vi "Calculate Jacobian.vi"(7 "Error Evaluation":T6, 9 "Validation Set":T2[](array[typedef]), 10 "Teaching Set":T2[](array[typedef]), 11 "Neural Network In":T4) -> (2 "Total Error":dbl, 3 "Jacobian":T1[][](array[typedef]))   [LabVIEW 2011, in "Super Simple Neural Network.lvlib"]
uses:
  Super Simple Neural Network.lvlib
  Types/Error Evaluation.ctl
  Types/2D Array.ctl
  Types/Neural Network.ctl
  Types/1D Array.ctl
  Types/Teaching Vector.ctl
  Types/Scaling Info.ctl
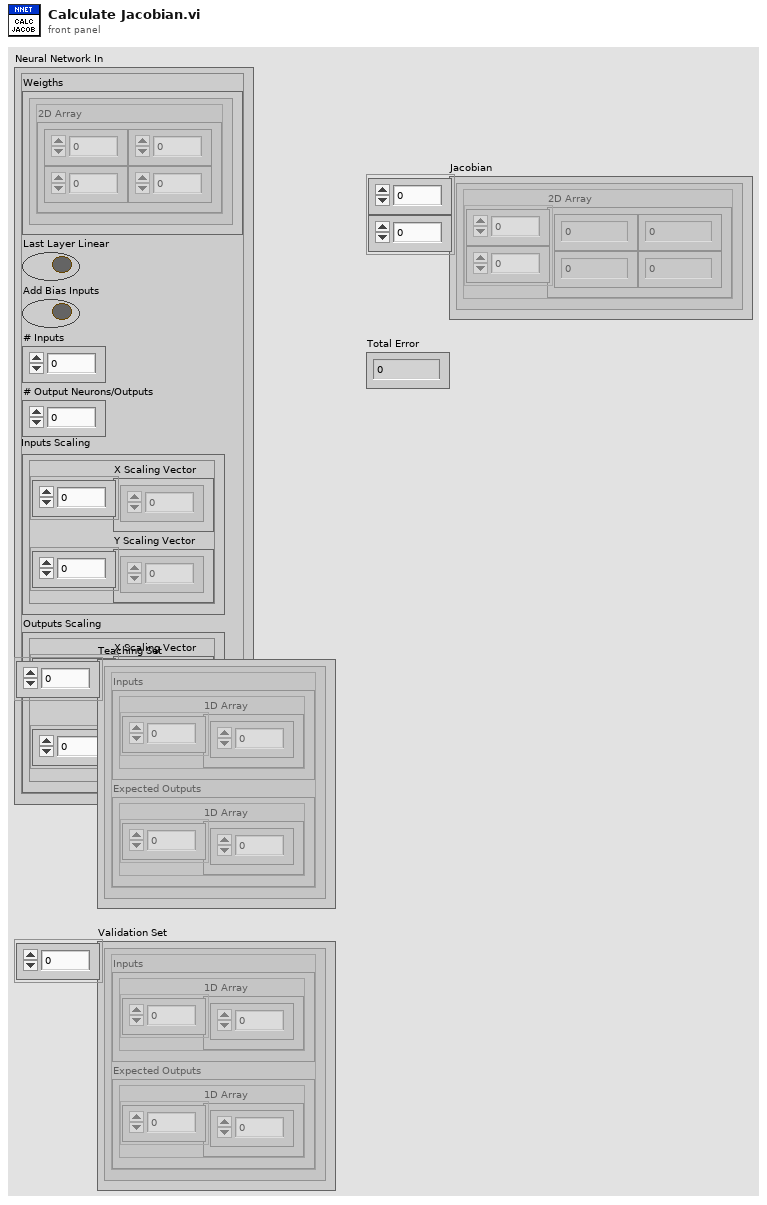
[diagram p1: front panel]
types:
  T1 = typedef "Super Simple Neural Network.lvlib/2D Array.ctl" = cluster{"2D Array":dbl[][]}
  T2 = typedef "Super Simple Neural Network.lvlib/Teaching Vector.ctl" = cluster{"Inputs":T3, "Expected Outputs":T3}
  T3 = typedef "Super Simple Neural Network.lvlib/1D Array.ctl" = cluster{"1D Array":dbl[]}
  T4 = typedef "Super Simple Neural Network.lvlib/Neural Network.ctl" = cluster{"Weigths":T1[], "Last Layer Linear":bool, "Add Bias Inputs":bool, "# Inputs":u32, "# Output Neurons/Outputs":u32, "Inputs Scaling":T5, "Outputs Scaling":T5}
  T5 = typedef "Super Simple Neural Network.lvlib/Scaling Info.ctl" = cluster{"X Scaling Vector":dbl[], "Y Scaling Vector":dbl[]}
  T6 = typedef "Super Simple Neural Network.lvlib/Error Evaluation.ctl" = enum16{"Over Both Sets", "Over Validation Set", "Over Teaching Set"}
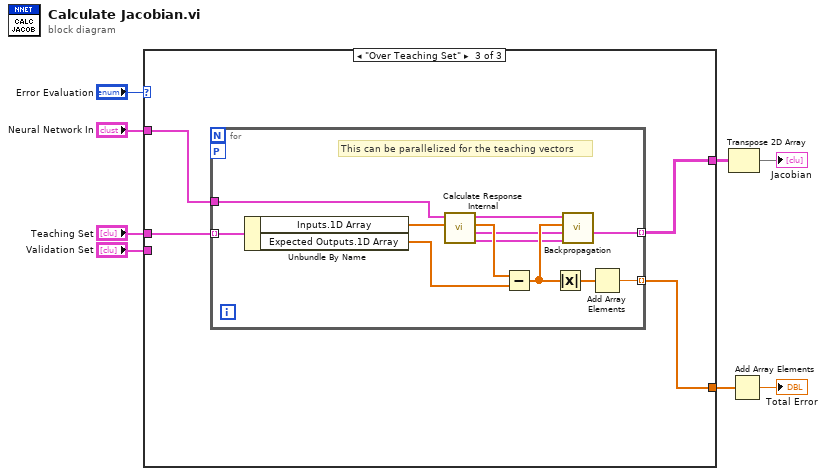
[diagram p0: block diagram]
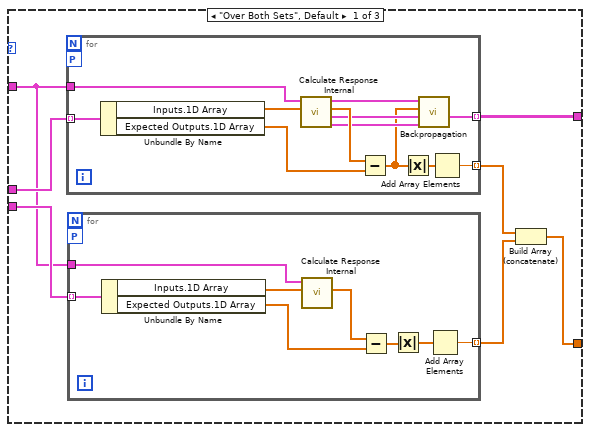
[diagram p2: hidden frame]
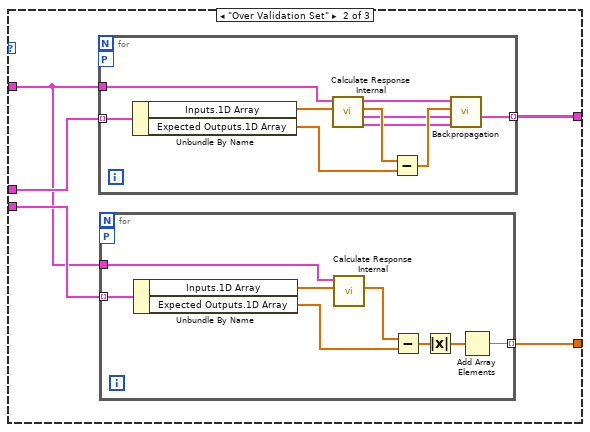
[diagram p3: hidden frame]
diagram:
  n1 = case shown="\"Over Teaching Set\"" "Error Evaluation" {
    tunnel: "Neural Network In" -> [w12 w37 w62]
    tunnel: "Teaching Set" -> [w15 w40 w61]
    tunnel: [w9 w36 w60] -> w1
    tunnel: [w14 w39 w59] -> w3
    tunnel: "Validation Set" -> [w13 w38 _]
    frame "Over Both Sets", Default {
      n2 = for {
        tunnel: w15 -> [w35] mode=indexing
        tunnel: [w27] -> w14 mode=indexing
        workers-P: _ -> [_]
        tunnel: w12 -> [w31]
        tunnel: [w24] -> w11 mode=indexing
        n3 = Unbundle By Name(w35) -> ("Inputs.1D Array"=w33:dbl[], "Expected Outputs.1D Array"=w34:dbl[])
        n4 = call "Calculate Response Internal.vi"("Inputs"=w33, "Neural Network In"=w31) -> ("All Inputs"=w28:T3[], "Derrivatives"=w29:T3[], "Outputs"=w32:dbl[], "Neural Network Out"=w30:T4)  [unwired: 6 in]
        n5 = Subtract(x=w32, y=w34) -> (x-y=w25:dbl[])
        n6 = Absolute Value(x=w25) -> (abs(x)=w26:dbl[])
        n7 = call "Backpropagation.vi"("All Inputs"=w28, "Derrivatives"=w29, "Error"=w25, "Neural Network In"=w30) -> ("Gradient Out"=w27:T1[])  [unwired: 7 in]
        n8 = Add Array Elements(numeric array=w26) -> (sum=w24:dbl)
      }
      n9 = for {
        tunnel: w13 -> [w23] mode=indexing
        workers-P: _ -> [_]
        tunnel: w12 -> [w19]
        tunnel: [w16] -> w10 mode=indexing
        n10 = Unbundle By Name(w23) -> ("Inputs.1D Array"=w21:dbl[], "Expected Outputs.1D Array"=w22:dbl[])
        n11 = call "Calculate Response Internal.vi"("Inputs"=w21, "Neural Network In"=w19) -> ("Outputs"=w20:dbl[])  [unwired: 6 in, 3 out]
        n12 = Subtract(x=w20, y=w22) -> (x-y=w17:dbl[])
        n13 = Absolute Value(x=w17) -> (abs(x)=w18:dbl[])
        n14 = Add Array Elements(numeric array=w18) -> (sum=w16:dbl)
      }
      n15 = Build Array (concatenate)(w11, w10) -> (w9:dbl[])
    }
    frame "Over Validation Set" {
      n16 = for {
        tunnel: w40 -> [w58] mode=indexing
        tunnel: [w49] -> w39 mode=indexing
        workers-P: _ -> [_]
        tunnel: w37 -> [w54]
        n17 = Unbundle By Name(w58) -> ("Inputs.1D Array"=w56:dbl[], "Expected Outputs.1D Array"=w57:dbl[])
        n18 = call "Calculate Response Internal.vi"("Inputs"=w56, "Neural Network In"=w54) -> ("All Inputs"=w50:T3[], "Derrivatives"=w51:T3[], "Outputs"=w55:dbl[], "Neural Network Out"=w53:T4)  [unwired: 6 in]
        n19 = Subtract(x=w55, y=w57) -> (x-y=w52:dbl[])
        n20 = call "Backpropagation.vi"("All Inputs"=w50, "Derrivatives"=w51, "Error"=w52, "Neural Network In"=w53) -> ("Gradient Out"=w49:T1[])  [unwired: 7 in]
      }
      n21 = for {
        tunnel: w38 -> [w48] mode=indexing
        workers-P: _ -> [_]
        tunnel: w37 -> [w44]
        tunnel: [w41] -> w36 mode=indexing
        n22 = Unbundle By Name(w48) -> ("Inputs.1D Array"=w46:dbl[], "Expected Outputs.1D Array"=w47:dbl[])
        n23 = call "Calculate Response Internal.vi"("Inputs"=w46, "Neural Network In"=w44) -> ("Outputs"=w45:dbl[])  [unwired: 6 in, 3 out]
        n24 = Subtract(x=w45, y=w47) -> (x-y=w42:dbl[])
        n25 = Absolute Value(x=w42) -> (abs(x)=w43:dbl[])
        n26 = Add Array Elements(numeric array=w43) -> (sum=w41:dbl)
      }
    }
    frame "Over Teaching Set" {
      n27 = for {
        tunnel: w61 -> [w74] mode=indexing
        tunnel: [w64] -> w59 mode=indexing
        workers-P: _ -> [_]
        tunnel: [w68] -> w60 mode=indexing
        tunnel: w62 -> [w70]
        # "This can be parallelized for the teaching vectors"
        n28 = Unbundle By Name(w74) -> ("Inputs.1D Array"=w72:dbl[], "Expected Outputs.1D Array"=w73:dbl[])
        n29 = call "Calculate Response Internal.vi"("Inputs"=w72, "Neural Network In"=w70) -> ("All Inputs"=w65:T3[], "Derrivatives"=w66:T3[], "Outputs"=w71:dbl[], "Neural Network Out"=w63:T4)  [unwired: 6 in]
        n30 = Subtract(x=w71, y=w73) -> (x-y=w67:dbl[])
        n31 = Absolute Value(x=w67) -> (abs(x)=w69:dbl[])
        n32 = call "Backpropagation.vi"("All Inputs"=w65, "Derrivatives"=w66, "Error"=w67, "Neural Network In"=w63) -> ("Gradient Out"=w64:T1[])  [unwired: 7 in]
        n33 = Add Array Elements(numeric array=w69) -> (sum=w68:dbl)
      }
    }
  }
  n34 = Transpose 2D Array(2D array=w3) -> (transposed array=→"Jacobian":T1[][])
  n35 = Add Array Elements(numeric array=w1) -> (sum=→"Total Error":dbl)
